vi "Teleop.vi"(10 "Match Info":T1={"Autonomous Elapsed Seconds"=0.0, "TeleOp Elapsed Seconds"=0.0, "Disabled Elapsed Seconds"=0.0, "Visited Autonomous"=FALSE, "Visited TeleOp"=FALSE, "Visited Disabled"=FALSE, "Autonomous Settings"={"Autonomous Style"=enum."Independent", "VI Refnum"=refnum}}, 11 "Call Context":T2) -> ()   [LabVIEW 2019]
doc: "This VI is called for each enabled TeleOp packet received from the DS. It is typically used to read from joysticks and other inputs and update I/O or setpoints for timed control loops. It should complete and return within 20 milliseconds or risk missing DS packets."
uses:
  <vilib>/Rock Robotics/WPI/DriverStation/WPI_DriverStationDerivedRobotMode.ctl
  <vilib>/Rock Robotics/WPI/DriverStation/WPI_DriverStationMatch Info.ctl
  Framework/Robot Global Data.vi
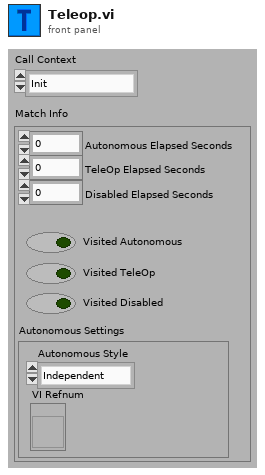
[diagram p1: front panel]
types:
  T1 = typedef "WPI_DriverStationMatch Info.ctl" = cluster{"Autonomous Elapsed Seconds":dbl, "TeleOp Elapsed Seconds":dbl, "Disabled Elapsed Seconds":dbl, "Visited Autonomous":bool, "Visited TeleOp":bool, "Visited Disabled":bool, "Autonomous Settings":cluster{"Autonomous Style":enum16{"Iterative", "Independent"}, "VI Refnum":refnum<vi>}}
  T2 = typedef "WPI_DriverStationDerivedRobotMode.ctl" = enum16{"Init", "Execute", "Stop"}
  T3 = typedef "Command Status Info.ctl" = cluster{"Name":string, "Status":T4, "notifier out":T5}
  T4 = typedef "Completion Status.ctl" = enum16{"Successful", "Aborted", "Incomplete"}
  T5 = typedef "Completion Notifier.ctl" = refnum<notifier>
  T6 = enum16{"Pipeline 0", "Pipeline 1", "Pipeline 2", "Pipeline 3", "Pipeline 4", "Pipeline 5", "Pipeline 6", "Pipeline 7", "Pipeline 8", "Pipeline 9"}
  T7 = cluster{"XAngle":dbl, "YAngle":dbl, "ZAngle":dbl}
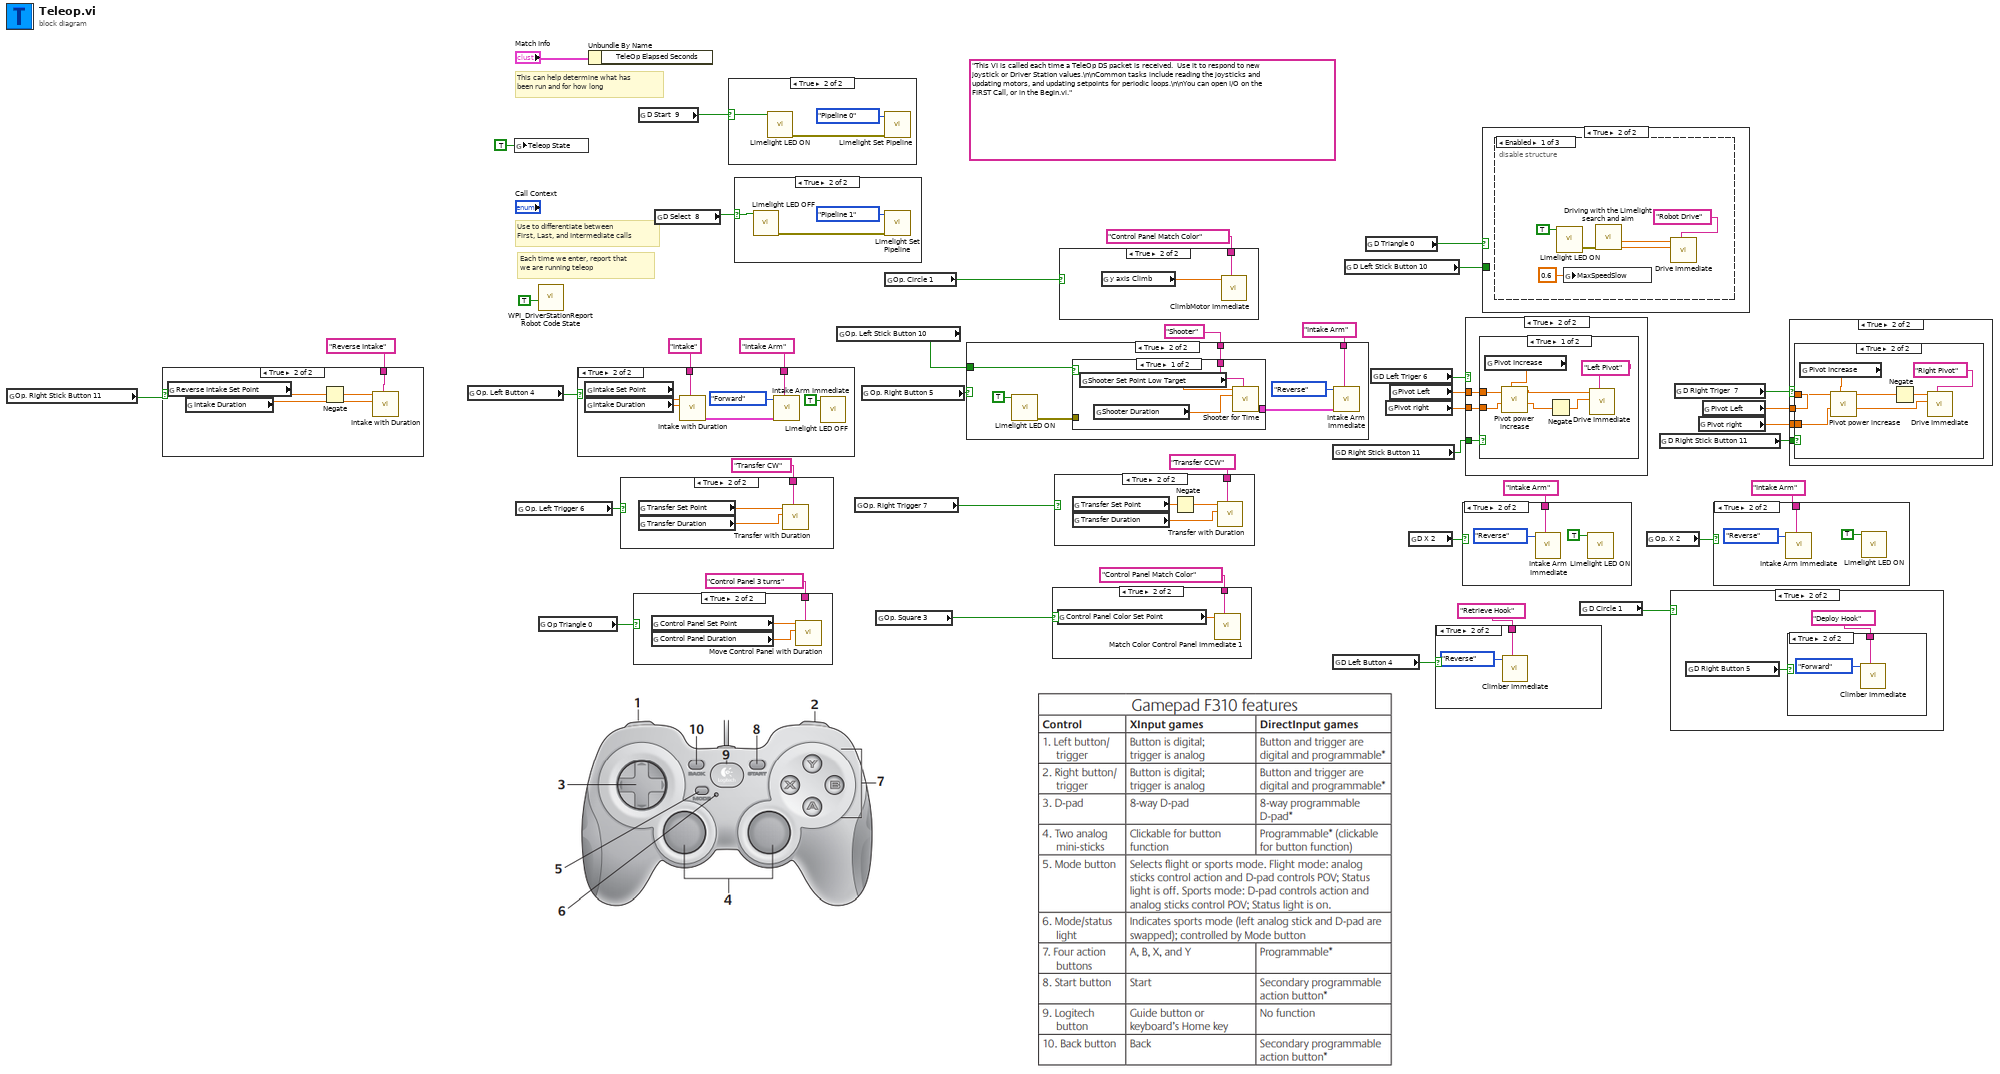
[diagram p0: block diagram]
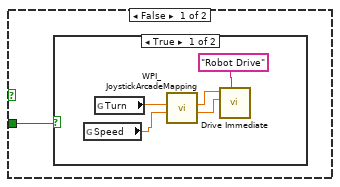
[diagram p10: hidden frame]
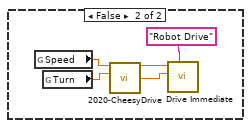
[diagram p11: hidden frame]
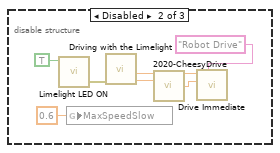
[diagram p12: hidden frame]
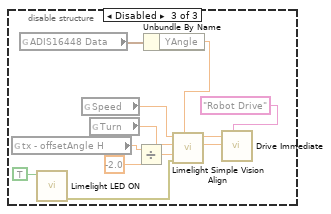
[diagram p13: hidden frame]
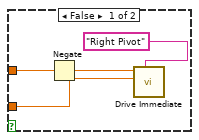
[diagram p18: hidden frame]
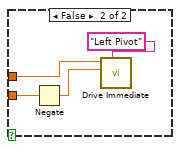
[diagram p20: hidden frame]
diagram:
  (unwired) "This VI is called each time a TeleOp DS packet is received.  Use it to respond to new joystick or Driver Station values.\n\nCommon tasks include reading the joysticks and updating motors, and updating setpoints for periodic loops.\n\nYou can open I/O on the FIRST Call, or in the Begin.vi."
  # "Each time we enter, report that\nwe are running teleop"
  # "Use to differentiate between\nFirst, Last, and Intermediate calls"
  # "This can help determine what has\nbeen run and for how long"
  n1 = global read "Robot Global Data.vi" "Op. Right Stick Button 11"() -> (w4:bool)
  n2 = case shown="True" w4 {
    tunnel: "Reverse Intake" ("refnum name") -> [_ w45]
    frame False {
    }
    frame True {
      n3 = global read "Robot Global Data.vi" "Reverse Intake Set Point"() -> (w44:dbl)
      n4 = global read "Robot Global Data.vi" "Intake Duration"() -> (w43:dbl)
      n5 = Negate(x=w44) -> (-x=w42:dbl)
      n6 = call "Intake with Duration.vi"("Description"=w45, "Duration (s)"=w43, "Setpoint"=w42) -> ()  [unwired: 8 in, 1 out]
    }
  }
  n7 = global read "Robot Global Data.vi" "Op. Left Button 4"() -> (w39:bool)
  n8 = global write "Robot Global Data.vi" "Teleop State"(TRUE ("Teleop State")) -> ()
  n9 = global read "Robot Global Data.vi" "Op. Left Trigger 6"() -> (w33:bool)
  n10 = call <vilib>:"WPI_DriverStationReport Robot Code State.vi"("TeleOp"=TRUE ("Autonomous")) -> ()  [unwired: 10 in, 1 out]
  n11 = global read "Robot Global Data.vi" "Op Triangle 0"() -> (w26:bool)
  n12 = case shown="True" w39 {
    tunnel: "Intake" ("refnum name") -> [_ w52]
    tunnel: "Intake Arm" ("refnum name") -> [_ w48]
    frame False {
    }
    frame True {
      n13 = global read "Robot Global Data.vi" "Intake Set Point"() -> (w51:dbl)
      n14 = global read "Robot Global Data.vi" "Intake Duration"() -> (w50:dbl)
      n15 = call "Intake with Duration.vi"("Description"=w52, "Duration (s)"=w50, "Setpoint"=w51) -> ("Command Info Out"=w47:T3)  [unwired: 8 in]
      n16 = call "Intake Arm Immediate.vi"("Description"=w48, "Command Info In"=w47, "Relay Value"=enum16{"Off", "On", "Forward", "Reverse"}."Forward") -> ()  [unwired: 8 in, 1 out]
      n17 = call "Limelight LED OFF.vi"("D Select  8"=TRUE) -> ()  [unwired: 10 in, 1 out]
    }
  }
  n18 = Unbundle By Name("Match Info") -> ()  [unwired: 1 out]
  n19 = case shown="True" w33 {
    tunnel: "Transfer CW" ("refnum name") -> [_ w55]
    frame False {
    }
    frame True {
      n20 = global read "Robot Global Data.vi" "Transfer Set Point"() -> (w54:dbl)
      n21 = global read "Robot Global Data.vi" "Transfer Duration"() -> (w53:dbl)
      n22 = call "Transfer with Duration.vi"("Description"=w55, "Duration (s)"=w53, "Setpoint"=w54) -> ()  [unwired: 8 in, 1 out]
    }
  }
  n23 = case shown="True" w26 {
    tunnel: "Control Panel 3 turns" ("refnum name") -> [_ w58]
    frame False {
    }
    frame True {
      n24 = global read "Robot Global Data.vi" "Control Panel Set Point"() -> (w57:dbl)
      n25 = global read "Robot Global Data.vi" "Control Panel Duration"() -> (w56:dbl)
      n26 = call "Move Control Panel with Duration.vi"("Description"=w58, "Duration (s)"=w56, "Setpoint"=w57) -> ()  [unwired: 8 in, 1 out]
    }
  }
  n27 = global read "Robot Global Data.vi" "D Start  9"() -> (w2:bool)
  n28 = global read "Robot Global Data.vi" "D Select  8"() -> (w1:bool)
  n29 = case shown="True" w2 {
    selector: w2 -> [_ w59]
    frame False {
    }
    frame True {
      n30 = call "Limelight LED ON.vi"("D Start  9"=w59) -> ("error out"=w61:errorcluster)  [unwired: 10 in]
      n31 = call "Limelight Set Pipeline.vi"("error in (no error)"=w61, "Pipeline number"=T6."Pipeline 0") -> ()  [unwired: 9 in, 1 out]
    }
  }
  n32 = case shown="True" w1 {
    selector: w1 -> [_ w64]
    frame False {
    }
    frame True {
      n33 = call "Limelight LED OFF.vi"("D Select  8"=w64) -> ("error out"=w62:errorcluster)  [unwired: 10 in]
      n34 = call "Limelight Set Pipeline.vi"("error in (no error)"=w62, "Pipeline number"=T6."Pipeline 1") -> ()  [unwired: 9 in, 1 out]
    }
  }
  n35 = global read "Robot Global Data.vi" "Op. Left Stick Button 10"() -> (w9:bool)
  n36 = global read "Robot Global Data.vi" "Op. Right Trigger 7"() -> (w34:bool)
  n37 = global read "Robot Global Data.vi" "Op. Right Button 5"() -> (w35:bool)
  n38 = global read "Robot Global Data.vi" "Op. Square 3"() -> (w23:bool)
  n39 = global read "Robot Global Data.vi" "Op. Circle 1"() -> (w11:bool)
  n40 = case shown="True" w35 {
    tunnel: "Shooter" ("refnum name") -> [_ w71]
    tunnel: "Intake Arm" ("refnum name") -> [_ w69]
    tunnel: w9 -> [_ w67]
    frame False {
    }
    frame True {
      n41 = call "Limelight LED ON.vi"("D Start  9"=TRUE) -> ("error out"=w65:errorcluster)  [unwired: 10 in]
      n42 = case shown="True" w67 {
        tunnel: w71 -> [w75 w79]
        tunnel: [w72 w76] -> w68
        tunnel: w65 -> [_ _]
        frame True {
          n43 = global read "Robot Global Data.vi" "Shooter Set Point Low Target"() -> (w74:dbl)
          n44 = global read "Robot Global Data.vi" "Shooter Duration"() -> (w73:dbl)
          n45 = call "Shooter for Time.vi"("Description"=w75, "Duration (s)"=w73, "Setpoint"=w74) -> ("Command Info Out"=w72:T3)  [unwired: 8 in]
        }
        frame False {
          n46 = global read "Robot Global Data.vi" "Shooter Set Point"() -> (w78:dbl)
          n47 = global read "Robot Global Data.vi" "Shooter Duration"() -> (w77:dbl)
          n48 = call "Shooter for Time.vi"("Description"=w79, "Duration (s)"=w77, "Setpoint"=w78) -> ("Command Info Out"=w76:T3)  [unwired: 8 in]
        }
      }
      n49 = call "Intake Arm Immediate.vi"("Description"=w69, "Command Info In"=w68, "Relay Value"=enum16{"Off", "On", "Forward", "Reverse"}."Reverse") -> ()  [unwired: 8 in, 1 out]
    }
  }
  n50 = case shown="True" w23 {
    tunnel: "Control Panel Match Color" ("refnum name") -> [_ w81]
    frame False {
    }
    frame True {
      n51 = global read "Robot Global Data.vi" "Control Panel Color Set Point"() -> (w80:dbl)
      n52 = call "Match Color Control Panel Immediate 1.vi"("Description"=w81, "Setpoint"=w80) -> ()  [unwired: 9 in, 1 out]
    }
  }
  n53 = case shown="True" w34 {
    tunnel: "Transfer CCW" ("refnum name") -> [_ w85]
    frame False {
    }
    frame True {
      n54 = global read "Robot Global Data.vi" "Transfer Set Point"() -> (w83:dbl)
      n55 = global read "Robot Global Data.vi" "Transfer Duration"() -> (w82:dbl)
      n56 = Negate(x=w83) -> (-x=w84:dbl)
      n57 = call "Transfer with Duration.vi"("Description"=w85, "Duration (s)"=w82, "Setpoint"=w84) -> ()  [unwired: 8 in, 1 out]
    }
  }
  n58 = case shown="True" w11 {
    tunnel: "Control Panel Match Color" ("refnum name") -> [_ w87]
    frame False {
    }
    frame True {
      n59 = global read "Robot Global Data.vi" "y axis Climb"() -> (w86:dbl)
      n60 = call "ClimbMotor Immediate.vi"("Description"=w87, "Setpoint"=w86) -> ()  [unwired: 9 in, 1 out]
    }
  }
  n61 = global read "Robot Global Data.vi" "D Right Stick Button 11"() -> (w6:bool)
  n62 = global read "Robot Global Data.vi" "D Left Button 4"() -> (w16:bool)
  n63 = global read "Robot Global Data.vi" "D Left Stick Button 10"() -> (w8:bool)
  n64 = global read "Robot Global Data.vi" "D Triangle 0"() -> (w17:bool)
  n65 = global read "Robot Global Data.vi" "D Left Triger 6"() -> (w31:bool)
  n66 = global read "Robot Global Data.vi" "Pivot right"() -> (w20:dbl)
  n67 = global read "Robot Global Data.vi" "Pivot Left"() -> (w21:dbl)
  n68 = global read "Robot Global Data.vi" "D X 2"() -> (w24:bool)
  n69 = case shown="True" w16 {
    tunnel: "Retrieve Hook" ("refnum name") -> [_ w88]
    frame False {
    }
    frame True {
      n70 = call "Climber Immediate.vi"("Description"=w88, "Value"=enum16{"Off", "On", "Forward", "Reverse"}."Reverse" ("Relay Value")) -> ()  [unwired: 9 in, 1 out]
    }
  }
  n71 = case shown="True" w24 {
    tunnel: "Intake Arm" ("refnum name") -> [_ w91]
    frame False {
    }
    frame True {
      n72 = call "Intake Arm Immediate.vi"("Description"=w91, "Relay Value"=enum16{"Off", "On", "Forward", "Reverse"}."Reverse") -> ()  [unwired: 9 in, 1 out]
      n73 = call "Limelight LED ON.vi"("D Start  9"=TRUE) -> ()  [unwired: 10 in, 1 out]
    }
  }
  n74 = case shown="True" w31 {
    tunnel: w21 -> [_ w95]
    tunnel: w20 -> [_ w94]
    tunnel: w6 -> [_ w93]
    frame False {
    }
    frame True {
      n75 = case shown="True" w93 {
        tunnel: w95 -> [w100 w105]
        tunnel: w94 -> [w99 w104]
        frame True {
          n76 = global read "Robot Global Data.vi" "Pivot Increase"() -> (w96:dbl)
          n77 = call "Pivot power increase.vi"("Pivot Increase"=w96, "Input Pivot Right"=w99, "Input Pivot Left"=w100) -> ("Output Pivot Right"=w97:dbl, "Output Pivot Left"=w98:dbl)  [unwired: 7 in]
          n78 = Negate(x=w97) -> (-x=w101:dbl)
          n79 = call "Drive Immediate.vi"("Description"="Left Pivot", "Right Setpoint"=w101, "Left Setpoint"=w98) -> ()  [unwired: 8 in, 1 out]
        }
        frame False {
          n80 = Negate(x=w104) -> (-x=w103:dbl)
          n81 = call "Drive Immediate.vi"("Description"="Left Pivot", "Right Setpoint"=w103, "Left Setpoint"=w105) -> ()  [unwired: 8 in, 1 out]
        }
      }
    }
  }
  n82 = case shown="True" w17 {
    tunnel: w8 -> [w107 _]
    frame False {
      n83 = case shown="True" w107 {
        frame True {
          n84 = global read "Robot Global Data.vi" "Speed"() -> (w110:dbl)
          n85 = global read "Robot Global Data.vi" "Turn"() -> (w111:dbl)
          n86 = call <vilib>:"WPI_JoystickArcadeMapping.vi"("Y axis value"=w110, "X axis value"=w111) -> ("Right Motor Value"=w108:dbl, "Left Motor Value"=w109:dbl)  [unwired: 8 in]
          n87 = call "Drive Immediate.vi"("Description"="Robot Drive", "Right Setpoint"=w108, "Left Setpoint"=w109) -> ()  [unwired: 8 in, 1 out]
        }
        frame False {
          n88 = global read "Robot Global Data.vi" "Speed"() -> (w114:dbl)
          n89 = global read "Robot Global Data.vi" "Turn"() -> (w115:dbl)
          n90 = call "2020-CheesyDrive.vi"("Throttle"=w114, "Wheel"=w115) -> ("Left PWM"=w116:dbl, "Right PWM"=w117:dbl)  [unwired: 12 in]
          n91 = call "Drive Immediate.vi"("Description"="Robot Drive", "Right Setpoint"=w117, "Left Setpoint"=w116) -> ()  [unwired: 8 in, 1 out]
        }
      }
    }
    frame True {
      n92 = disable-structure shown="Enabled" {
        frame Enabled {
          n93 = call "Limelight LED ON.vi"("D Start  9"=TRUE) -> ("error out"=w122:errorcluster)  [unwired: 10 in]
          n94 = global write "Robot Global Data.vi" "MaxSpeedSlow"(0.6 ("MaxSpeedSlow")) -> ()
          n95 = call "Driving with the Limelight search and aim.vi"("error in (no error)"=w122) -> ("TurnCommand"=w118:dbl, "SpeedCommand"=w119:dbl)  [unwired: 8 in, 1 out]
          n96 = call "Drive Immediate.vi"("Description"="Robot Drive", "Right Setpoint"=w118, "Left Setpoint"=w119) -> ()  [unwired: 8 in, 1 out]
        }
        frame Disabled {
          n97 = call "Limelight LED ON.vi"("D Start  9"=TRUE) -> ("error out"=w126:errorcluster)  [unwired: 10 in]
          n98 = global write "Robot Global Data.vi" "MaxSpeedSlow"(0.6 ("MaxSpeedSlow")) -> ()
          n99 = call "Driving with the Limelight.vi"("error in (no error)"=w126) -> ("TurnCommand"=w127:dbl, "SpeedCommand"=w128:dbl)  [unwired: 8 in, 1 out]
          n100 = call "2020-CheesyDrive.vi"("Throttle"=w128, "Wheel"=w127) -> ("Left PWM"=w130:dbl, "Right PWM"=w131:dbl)  [unwired: 12 in]
          n101 = call "Drive Immediate.vi"("Description"="Robot Drive", "Right Setpoint"=w131, "Left Setpoint"=w130) -> ()  [unwired: 8 in, 1 out]
        }
        frame Disabled {
          n102 = global read "Robot Global Data.vi" "tx - offsetAngle H"() -> (w137:dbl)
          n103 = global read "Robot Global Data.vi" "ADIS16448 Data"() -> (w133:T7)
          n104 = call "Limelight LED ON.vi"("D Start  9"=TRUE) -> ("error out"=w141:errorcluster)  [unwired: 10 in]
          n105 = global read "Robot Global Data.vi" "Speed"() -> (w135:dbl)
          n106 = global read "Robot Global Data.vi" "Turn"() -> (w134:dbl)
          n107 = Divide(x=w137, y=-2.0) -> (x/y=w138:dbl)
          n108 = Unbundle By Name(w133) -> ("YAngle"=w132:dbl)
          n109 = call "Limelight Simple Vision Align.vi"("Gyro Angle"=w132, "error in (no error)"=w141, "Target Offset"=w138, "Manual Turn"=w134, "Throttle"=w135) -> ("Right Power"=w139:dbl, "Left Power"=w140:dbl)  [unwired: 5 in]
          n110 = call "Drive Immediate.vi"("Description"="Robot Drive", "Right Setpoint"=w139, "Left Setpoint"=w140) -> ()  [unwired: 8 in, 1 out]
        }
      }
    }
  }
  n111 = global read "Robot Global Data.vi" "D Circle 1"() -> (w10:bool)
  n112 = global read "Robot Global Data.vi" "Op. X 2"() -> (w14:bool)
  n113 = global read "Robot Global Data.vi" "D Right Stick Button 11"() -> (w7:bool)
  n114 = case shown="True" w10 {
    frame False {
    }
    frame True {
      n115 = global read "Robot Global Data.vi" "D Right Button 5"() -> (w144:bool)
      n116 = case shown="True" w144 {
        tunnel: "Deploy Hook" ("refnum name") -> [_ w146]
        frame False {
        }
        frame True {
          n117 = call "Climber Immediate.vi"("Description"=w146, "Value"=enum16{"Off", "On", "Forward", "Reverse"}."Forward" ("Relay Value")) -> ()  [unwired: 9 in, 1 out]
        }
      }
    }
  }
  n118 = global read "Robot Global Data.vi" "D Right Triger  7"() -> (w30:bool)
  n119 = global read "Robot Global Data.vi" "Pivot right"() -> (w18:dbl)
  n120 = global read "Robot Global Data.vi" "Pivot Left"() -> (w19:dbl)
  n121 = case shown="True" w14 {
    tunnel: "Intake Arm" ("refnum name") -> [_ w149]
    frame False {
    }
    frame True {
      n122 = call "Intake Arm Immediate.vi"("Description"=w149, "Relay Value"=enum16{"Off", "On", "Forward", "Reverse"}."Reverse") -> ()  [unwired: 9 in, 1 out]
      n123 = call "Limelight LED ON.vi"("D Start  9"=TRUE) -> ()  [unwired: 10 in, 1 out]
    }
  }
  n124 = case shown="True" w30 {
    tunnel: w19 -> [_ w153]
    tunnel: w18 -> [_ w152]
    tunnel: w7 -> [_ w151]
    frame False {
    }
    frame True {
      n125 = case shown="True" w151 {
        tunnel: w153 -> [w156 w162]
        tunnel: w152 -> [w155 w161]
        frame False {
          n126 = Negate(x=w156) -> (-x=w154:dbl)
          n127 = call "Drive Immediate.vi"("Description"="Right Pivot", "Right Setpoint"=w155, "Left Setpoint"=w154) -> ()  [unwired: 8 in, 1 out]
        }
        frame True {
          n128 = global read "Robot Global Data.vi" "Pivot Increase"() -> (w158:dbl)
          n129 = call "Pivot power increase.vi"("Pivot Increase"=w158, "Input Pivot Right"=w161, "Input Pivot Left"=w162) -> ("Output Pivot Right"=w159:dbl, "Output Pivot Left"=w160:dbl)  [unwired: 7 in]
          n130 = Negate(x=w160) -> (-x=w163:dbl)
          n131 = call "Drive Immediate.vi"("Description"="Right Pivot", "Right Setpoint"=w159, "Left Setpoint"=w163) -> ()  [unwired: 8 in, 1 out]
        }
      }
    }
  }
